vi "Test_WriteValue_InvalidRefnum_Error.vi"(8 "error in (no error)":errorcluster, 11 "TestCase in":refnum<class "TestBooleanTextBinding.lvclass">) -> (0 "error out":errorcluster, 3 "TestCase out":refnum<class "TestBooleanTextBinding.lvclass">)   [LabVIEW 2017, in "TestBooleanTextBinding.lvclass"]
uses:
  TestBooleanTextBinding.lvclass
  Source/Concrete/BooleanTextBinding/BooleanTextBinding.lvclass/BooleanTextBinding.ctl
  Source/Concrete/BooleanTextBinding/BooleanTextBinding.lvclass
  C:/Git/composed-transport/Source/ITransport/ITransport.lvclass
  <vilib>/Utility/error.llb/Error Cluster From Error Code.vi
  Source/ITransport/ITransport.lvclass
panel:
  out "Return Error":errorcluster
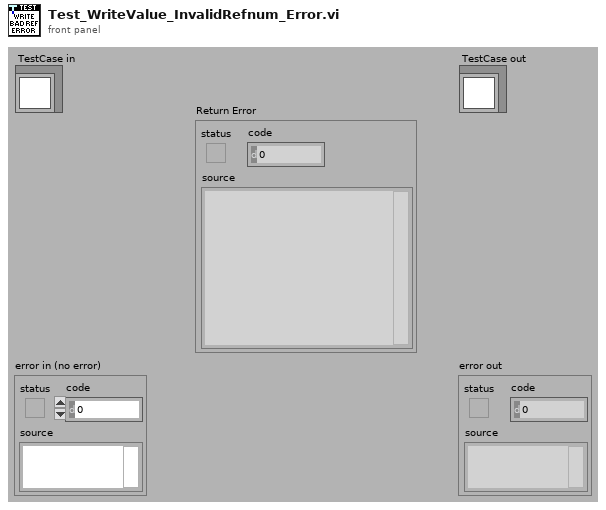
[diagram p1: front panel]
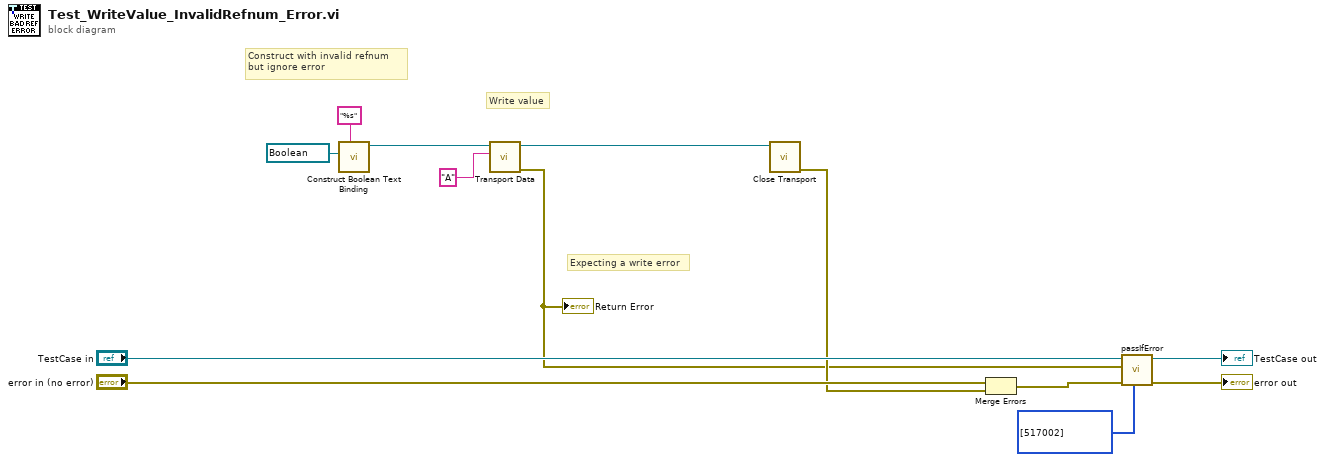
[diagram p0: block diagram]
diagram:
  # "Expecting a write error"
  # "Construct with invalid refnum\nbut ignore error"
  # "Write value"
  n1 = call "Construct Boolean Text Binding.vi"("Format String"="%s", "Bool Refnum"=refnum<vi> refnum) -> ("BooleanTextBinding"=w9:refnum<class "BooleanTextBinding.lvclass">)  [unwired: 8 in, 1 out]
  n2 = call "Transport Data.vi"("Value"="A" ("Format String"), "ITransport in"=w9) -> ("error out"=w3:errorcluster, "ITransport out"=w7:refnum<class "BooleanTextBinding.lvclass">)  [unwired: 8 in]
  "Return Error" <- w3
  n3 = call-dynamic "Close Transport.vi"("ITransport in"=w7) -> ("error out"=w6:errorcluster)  [unwired: 10 in]
  n4 = Merge Errors("error in (no error)", w6) -> (w8:errorcluster)
  n5 = call-dynamic "passIfError.vi"("passing error codes (default = any error code)"=i32[] [517002], "error in (no error)"=w8, "error"=w3, "TestCase in"="TestCase in") -> ("error out"=→"error out":errorcluster, "TestCase out"=→"TestCase out":refnum<class "TestBooleanTextBinding.lvclass">)  [unwired: 6 in]
